vi "Begin.vi"(8 "error in":errorcluster) -> (0 "error out":errorcluster)   [LabVIEW 2014]
doc: "Called before other user functions, this VI is expected to open initial I/O refnums, load in file data, and do all program initialization. Notice that the <B>error out</B> terminal is simply used for data flow. Wiring it to other structures or subVIs ensures that this VI runs first."
uses:
  <vilib>/Rock Robotics/WPI/DriverStation/WPI_DriverStationRobotMode2.ctl
  <vilib>/Rock Robotics/WPI/Joystick/WPI_JoystickDeviceEnum.ctl
  <vilib>/Rock Robotics/WPI/CAN/TalonSRX/WPI_CANTalonSRX_APIControlMode.ctl
  <vilib>/Rock Robotics/WPI/SafetyOutput/WPI_SafetyOutputConfigMenu.ctl
  <vilib>/Rock Robotics/WPI/Solenoid/WPI_SolenoidChannel.ctl
  navx-mxp/labview/navX-MXP Library/COMMON/TypeDefs/Value TypeDefs/navX Interface Protocol.ctl
  <vilib>/Rock Robotics/SystemInterfaces/spilib/spi_bus.ctl
  Robot Global Data.vi
  <vilib>/Rock Robotics/WPI/Solenoid/WPI_SolenoidOpenSingle.vi
  <vilib>/Rock Robotics/WPI/Compressor/WPI_CompressorGetSetRefNum.vi
  navx-mxp/labview/navX-MXP Library/navX-MXP IMU.lvlib
panel:
  out "Opened?":bool
  # "PID Options For Arm"
  # "RobotDrive Layout"
  # "PID Options for the Robot Drive"
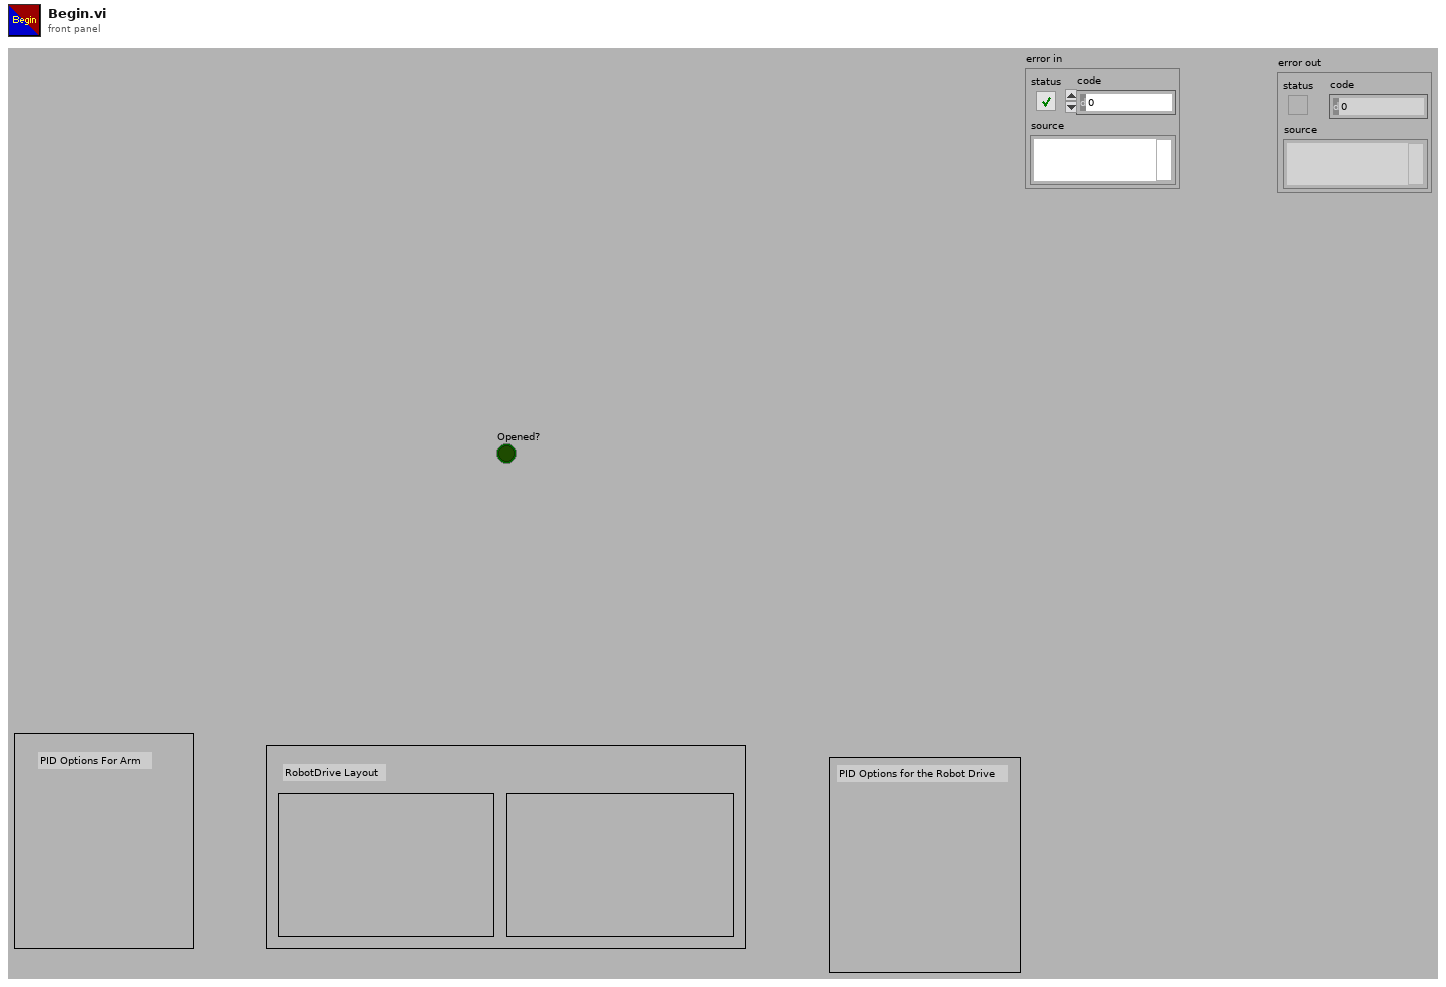
[diagram p1: front panel]
types:
  T1 = typedef "spi_bus.ctl" = enum16{"SPI On-Board, CS0", "SPI On-Board, CS1", "SPI On-Board, CS2", "SPI On-Board, CS3", "SPI MXP", "Invalid"}
  T2 = typedef "navX-MXP IMU.lvlib/navX Interface Protocol.ctl" = enum16{"SPI", "I2C", "SERIAL"}
  T3 = typedef "WPI_SolenoidChannel.ctl" = enum8{"Solenoid 0", "Solenoid 1", "Solenoid 2", "Solenoid 3", "Solenoid 4", "Solenoid 5", "Solenoid 6", "Solenoid 7", "Invalid"}
  T4 = typedef "WPI_SafetyOutputConfigMenu.ctl" = enum16{"Enable", "Disable"}
  T5 = typedef "WPI_CANTalonSRX_APIControlMode.ctl" = enum8{"Percent VBus", "Speed", "Position", "Slave", "Unchanged / Invalid"}
  T6 = typedef "WPI_JoystickDeviceEnum.ctl" = enum16{"USB 0", "USB 1", "USB 2", "USB 3", "USB 4", "USB 5"}
  T7 = typedef "WPI_DriverStationRobotMode2.ctl" = enum16{"Autonomous Disabled", "Autonomous Enabled", "Teleop Disabled", "Teleop Enabled", "Disconnected", "Finish", "Test Disabled", "Test Enabled", "Emergency Stopped"}
  T8 = typedef "navX-MXP IMU.lvlib/navX Device TypeDef.ctl" = cluster{"navX Interface Protocol":T2, "navX Interface Protocol TypeDefs":cluster{"SPIDevRef":T9, "I2CDevRef":T11}, "navX System Information":cluster{"Board Information":T13, "Status":T16, "Offsets":T20, "LastSampleTimestamp":dbl, "LastSampleValid":bool}, "navX Common Information":cluster{"Update Rate (4Hz-60Hz)":T21, "refnum name":string, "error":errorcluster, "LastSampleFPGATimestamp":dbl}}
  T9 = typedef "WPI_SPIDevRef.ctl" = cluster{"DevStatus":errorcluster, "Handle":i32, "Controller":T10, "SPI Bus":T1}
  T10 = typedef "FPGA_TypedefDigitalModule.ctl" = enum16{"Controller 1"}
  T11 = typedef "WPI_I2CDevRef.ctl" = cluster{"DevStatus":errorcluster, "Controller":T10, "Device Address":u8, "Handle":i32, "I2C Bus":T12}
  T12 = typedef "i2c_bus.ctl" = enum16{"I2C On-Board", "I2C MXP", "Invalid"}
  T13 = typedef "navX-MXP IMU.lvlib/navX Board Information.ctl" = cluster{"WhoAmI (50 | 0x32)":u8, "Board Revision":u8, "Firmware Major Version":u8, "Firmware Minor Version":u8, "NAVX_BOARD_CAPABILITY":T14, "NAVX_BOARD_YAW_AXIS":T15}
  T14 = typedef "navX-MXP IMU.lvlib/navX NAVX_BOARD_CAPABILITY.ctl" = cluster{"OMNIMOUNT":bool, "YAW_RESET":bool, "VEL_AND_DISP":bool}
  T15 = typedef "navX-MXP IMU.lvlib/navX NAVX_BOARD_YAW_AXIS.ctl" = cluster{"BOARD_YAW_AXIS_UP":bool, "BOARD_YAW_AXIS":u8}
  T16 = typedef "navX-MXP IMU.lvlib/navX Status Data.ctl" = cluster{"Update Rate Hz":u8, "Accelerometer Full-Scale Range":u8, "Gyro Full-Scale Range":u16, "NAVX_OP_STATUS":T17, "NAVX_CAL_STATUS":T18, "NAVX_SELFTEST_STATUS":u8, "NAVX_SENSOR_STATUS":T19}
  T17 = typedef "navX-MXP IMU.lvlib/navX NAVX_OP_STATUS.ctl" = u8
  T18 = typedef "navX-MXP IMU.lvlib/navX NAVX_CAL_STATUS.ctl" = u8
  T19 = typedef "navX-MXP IMU.lvlib/navX NAVX_SENSOR_STATUS.ctl" = cluster{"MOVING":bool, "YAW_STABLE":bool, "MAG_DISTURBANCE":bool, "ALTITUDE_VALID":bool, "SEALEVEL_PRESS_SET":bool, "FUSED_HEADING_VALID":bool}
  T20 = typedef "navX-MXP IMU.lvlib/navX Offsets Data.ctl" = cluster{"Yaw":dbl, "Quat W":dbl, "Quat X":dbl, "Quat Y":dbl, "Quat Z":dbl}
  T21 = typedef "navX-MXP IMU.lvlib/navX Update Rate.ctl" = u8
  T22 = typedef "WPI_MotorControlDeviceRef.ctl" = cluster{"DeviceStatus":errorcluster, "Type":T23, "PWM":cluster{"Controller":T10, "PWM Channel":T24, "DeadBand":T25}, "CAN":cluster{"Device Number":u8, "Control Mode":T26, "Semaphore":T27, "Max Vout":dbl, "TalonSRX Control Mode":T5}, "Invert":bool, "TransformRef":T28, "InvTransformRef":T28}
  T23 = typedef "WPI_MotorControlType.ctl" = enum16{"PWM", "CAN", "CANTalonSRX"}
  T24 = typedef "FPGA_DIOPWMChannel.ctl" = enum8{"PWM 0", "PWM 1", "PWM 2", "PWM 3", "PWM 4", "PWM 5", "PWM 6", "PWM 7", "PWM 8", "PWM 9", "PWM MXP 0", "PWM MXP 1", "PWM MXP 2", "PWM MXP 3", "PWM MXP 4", "PWM MXP 5", "PWM MXP 6", "PWM MXP 7", "PWM MXP 8", "PWM MXP 9", "Invalid"}
  T25 = typedef "WPI_PWMDeadband.ctl" = cluster{"Name":string, "maxPositivePwm":i32, "minPositivePwm":i32, "centerPwm":i32, "maxNegativePwm":i32, "minNegativePwm":i32, "angularRange":u16}
  T26 = typedef "WPI_CANJaguar_ControlMode.ctl" = enum8{"Percent VBus", "Current", "Speed", "Position", "Voltage"}
  T27 = typedef "Semaphore RefNum" = refnum<k1>
  T28 = typedef "WPI_PWMTransform_ConPane.ctl" = refnum<vi>
  T29 = typedef "WPI_CompressorDevRef.ctl" = cluster{"DevStatus":errorcluster, "Pneumatics Control Module":u8}
  T30 = typedef "WPI_SolenoidDevRef.ctl" = cluster{"DevStatus":errorcluster, "Pneumatics Control Module":u8, "Forward Solenoid Channel":T3, "Reverse Solenoid Channel":T3}
  T31 = typedef "WPI_RobotDriveDevRef.ctl" = cluster{"DevStatus":errorcluster, "Motors[]":T22[], "Square Inputs":bool, "Max Output":dbl}
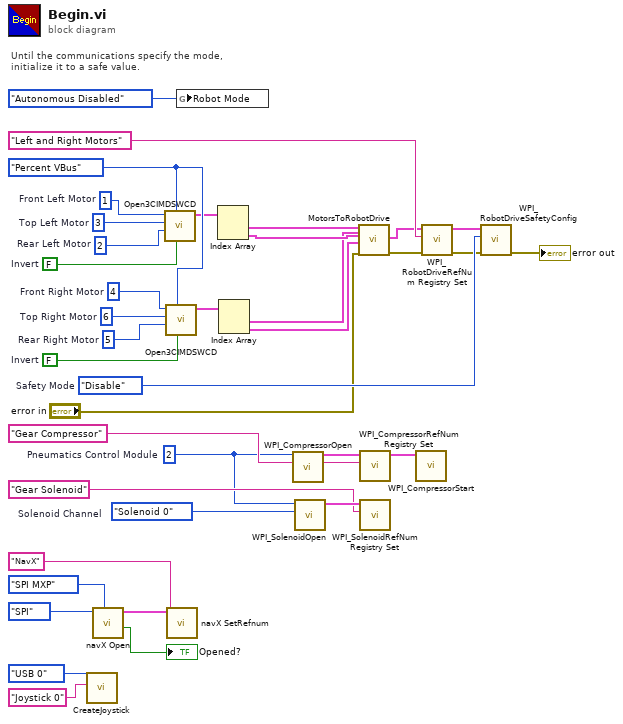
[diagram p0: block diagram]
diagram:
  w9 = FALSE  # Invert
  w1 = u8 2  # Pneumatics Control Module
  w28 = WPI_SolenoidChannel."Solenoid 0"  # Solenoid Channel
  w14 = FALSE  # Invert
  w11 = u8 6  # Top Right Motor
  w10 = u8 5  # Rear Right Motor
  w12 = u8 4  # Front Right Motor
  w16 = u8 3  # Top Left Motor
  w15 = u8 2  # Rear Left Motor
  w17 = u8 1  # Front Left Motor
  w35 = WPI_SafetyOutputConfigMenu."Disable"  # Safety Mode
  w13 = WPI_CANTalonSRX_APIControlMode."Percent VBus" ("Control Mode")
  # "Until the communications specify the mode,\ninitialize it to a safe value."
  n1 = call "CreateJoystick.vi"("refnum name"="Joystick 0", "JoystickDevice"=WPI_JoystickDeviceEnum."USB 0") -> ()  [unwired: 6 in, 2 out]
  n2 = call "navX Open.vi"("SPI Bus"=spi_bus."SPI MXP", "navX Interface Protocol"=navX_Interface_Protocol."SPI") -> ("Opened?"=→"Opened?":bool, "navX Device TypeDef"=w19:T8)  [unwired: 7 in, 1 out]
  n3 = call "Open3CIMDSWCD.vi"("Invert"=w14, "Control Mode"=w13, "Bottom Back"=w15, "Top Middle"=w16, "Bottom Front"=w17) -> ("Motor Instances"=w8:T22[])  [unwired: 6 in]
  n4 = call "Open3CIMDSWCD.vi"("Invert"=w9, "Control Mode"=w13, "Bottom Back"=w10, "Top Middle"=w11, "Bottom Front"=w12) -> ("Motor Instances"=w5:T22[])  [unwired: 6 in]
  n5 = call "navX SetRefnum.vi"("refnum name"="NavX", "navX Device TypeDef"=w19) -> ()  [unwired: 8 in, 2 out]
  n6 = global write "Robot Global Data.vi" "Robot Mode"(WPI_DriverStationRobotMode2."Autonomous Disabled" ("Robot Mode")) -> ()
  n7 = Index Array(array=w8) -> (element #1=w7:T22, element #2=w6:T22)  [unwired: 2 in]
  n8 = Index Array(array=w5) -> (element #1=w4:T22, element #2=w3:T22)  [unwired: 2 in]
  n9 = call <vilib>:"WPI_CompressorOpen.vi"("Pneumatics Control Module (0)"=w1) -> ("CompressorDevRef"=w27:T29)  [unwired: 13 in, 1 out]
  n10 = call-poly <vilib>:"WPI_SolenoidOpen.vi"("Solenoid Channel"=w28, "Pneumatics Control Module (0)"=w1) -> ("SolenoidDevRef"=w25:T30)  [unwired: 8 in, 1 out]
  n11 = call "MotorsToRobotDrive.vi"("Left Motor 1"=w7, "Right Motor 1"=w4, "Left Motor 2"=w6, "Right Motor 2"=w3, "error in"="error in") -> ("RobotDriveDevRef"=w30:T31, "error out"=w2:errorcluster)  [unwired: 13 in]
  n12 = call <vilib>:"WPI_CompressorRefNum Registry Set.vi"("refnum name"="Gear Compressor", "CompressorDevRef"=w27) -> ("CompressorDevRef"=w23:T29)  [unwired: 8 in, 1 out]
  n13 = call <vilib>:"WPI_SolenoidRefNum Registry Set.vi"("refnum name"="Gear Solenoid", "SolenoidDevRef"=w25) -> ()  [unwired: 8 in, 2 out]
  n14 = call <vilib>:"WPI_CompressorStart.vi"("CompressorDevRef"=w23) -> ()  [unwired: 9 in, 2 out]
  n15 = call <vilib>:"WPI_RobotDriveRefNum Registry Set.vi"("error in (no error)"=w2, "refnum name"="Left and Right Motors", "RobotDriveDevRef"=w30) -> ("error out"=w31:errorcluster, "RobotDriveDevRef"=w33:T31)  [unwired: 7 out]
  n16 = call <vilib>:"WPI_RobotDriveSafetyConfig.vi"("error in (no error)"=w31, "mode"=w35, "RobotDriveDevRef"=w33) -> ("error out"=→"error out":errorcluster)  [unwired: 7 in, 1 out]
